vi "Write String.vi"(8 "error in (no error)":errorcluster, 10 "String":string, 11 "Gen2 in":refnum<class "KDemoDerived.lvclass">) -> (0 "error out":errorcluster, 3 "Gen2 out":refnum<class "KDemoDerived.lvclass">)   [LabVIEW 2015, in "KDemoDerived.lvclass"]
uses:
  KDemoDerived.lvclass
  KDemoDerived.lvclass/KDemoDerived.ctl
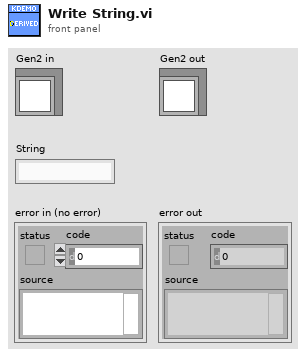
[diagram p1: front panel]
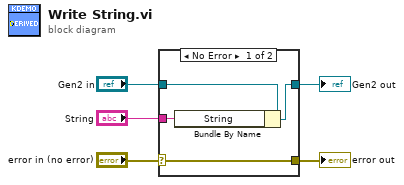
[diagram p0: block diagram]
diagram:
  n1 = case shown="No Error" "error in (no error)" {
    selector: "error in (no error)" -> [w9 w10]
    tunnel: [w9 w10] -> w4
    tunnel: [w7 w11] -> w2
    tunnel: "Gen2 in" -> [w8 w11]
    tunnel: "String" -> [w6 _]
    frame No Error {
      n2 = Bundle By Name(cluster=w8, "String"=w6) -> (w7:refnum<class "KDemoDerived.lvclass">)
    }
    frame Error {
    }
  }
  "error out" <- w4
  "Gen2 out" <- w2
